vi "create basic config.vi"(8 "error in":errorcluster) -> (0 "error out":errorcluster, 1 "instance identifier":string, 2 "generated channels":refnum<class "TBM channel.lvclass">[](array[class]), 3 "user tag bus module configuration out":refnum<class "user tag bus module configuration.lvclass">)   [LabVIEW 2013, in "user code tests.lvlib"]
uses:
  user code tests.lvlib
  module/configuration/user tag bus module configuration.lvclass
  <vilib>/NI/Tag Bus Module Framework/channel/TBM channel.lvclass
  <vilib>/NI/Configuration Framework/serializable configuration/NISE_CEF_serializable configuration.lvclass/NISE_CEF_serializable configuration.ctl
  <vilib>/NI/Configuration Framework/serializable configuration/NISE_CEF_serializable configuration.lvclass
  <vilib>/NI/Configuration Framework/serializable configuration/Read UID.vi
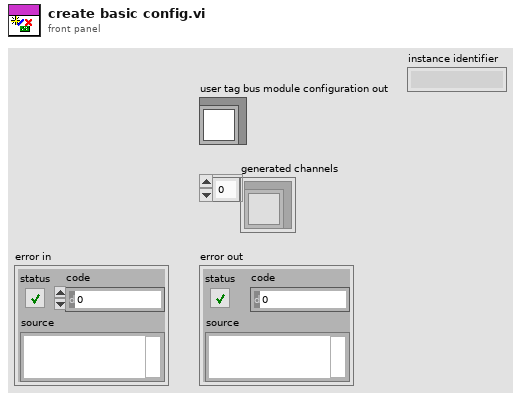
[diagram p1: front panel]
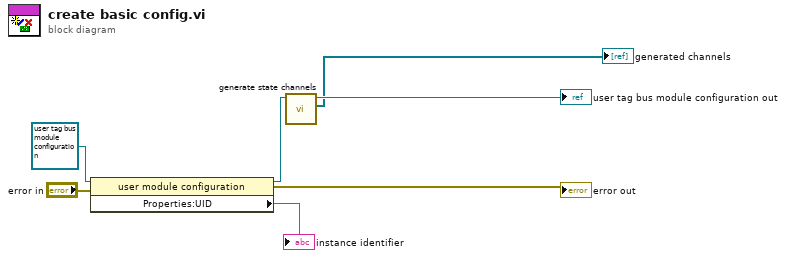
[diagram p0: block diagram]
diagram:
  n1 = property class="user module configuration"(reference=refnum<class "user tag bus module configuration.lvclass"> refnum ("tag bus configurable plugin module configuration"), error in="error in") -> (reference out=w4:refnum<class "user tag bus module configuration.lvclass">, error out=→"error out":errorcluster, "Properties:UID"=→"instance identifier":string)
  n2 = call "generate state channels.vi"("tag bus configurable plugin module configuration in"=w4) -> ("generated channels"=→"generated channels":refnum<class "TBM channel.lvclass">[], "tag bus configurable plugin module configuration out"=→"user tag bus module configuration out":refnum<class "user tag bus module configuration.lvclass">)  [unwired: 9 in]
